vi "FH5dataout.vi"() -> ()   [LabVIEW 2020]
uses:
  Velocimetro.ctl
  ContaGiro.ctl
panel:
  out "RPM x Speed":sgl[][](graph)
  out "Numeric 2":sgl format="%_4f"
  out "Numeric":sgl format="%_3g"
  out "Velocidade Km/h":T1 scale=0.0..300.0
  out "RPM":T2 scale=0.0..8.0
  in  "Stop Button":bool
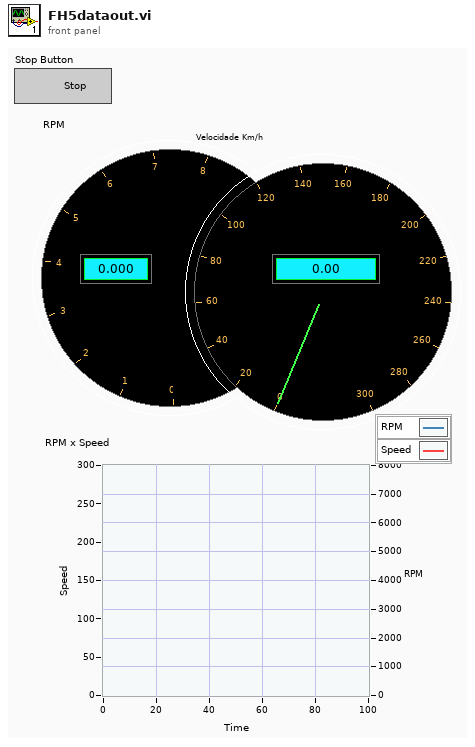
[diagram p1: front panel]
types:
  T1 = typedef "Velocimetro.ctl" = dbl
  T2 = typedef "ContaGiro.ctl" = dbl
  T3 = cluster{"IsRaceOn":i32, "TimestampMS":u32, "EngineMaxRpm":sgl, "EngineIdleRpm":sgl, "CurrentEngineRpm":sgl, "AccelerationX":sgl, "AccelerationY":sgl, "AccelerationZ":sgl, "VelocityX":sgl, "VelocityY":sgl, "VelocityZ":sgl, "AngularVelocityX":sgl, "AngularVelocityY":sgl, "AngularVelocityZ":sgl, "Yaw":sgl, "Pitch":sgl, "Roll":sgl, "NormalizedSuspensionTravelFrontLeft":sgl, "NormalizedSuspensionTravelFrontRight":sgl, "NormalizedSuspensionTravelRearLeft":sgl, "NormalizedSuspensionTravelRearRight":sgl, "TireSlipRatioFrontLeft":sgl, "TireSlipRatioFrontRight":sgl, "TireSlipRatioRearLeft":sgl, "TireSlipRatioRearRight":sgl, "WheelRotationSpeedFrontLeft":sgl, "WheelRotationSpeedFrontRight":sgl, "WheelRotationSpeedRearLeft":sgl, "WheelRotationSpeedRearRight":sgl, "WheelOnRumbleStripFrontLeft":i32, "WheelOnRumbleStripFrontRight":i32, "WheelOnRumbleStripRearLeft":i32, "WheelOnRumbleStripRearRight":i32, "WheelInPuddleDepthFrontLeft":sgl, "WheelInPuddleDepthFrontRight":sgl, "WheelInPuddleDepthRearLeft":sgl, "WheelInPuddleDepthRearRight":sgl, "SurfaceRumbleFrontLeft":sgl, "SurfaceRumbleFrontRight":sgl, "SurfaceRumbleRearLeft":sgl, "SurfaceRumbleRearRight":sgl, "TireSlipAngleFrontLeft":sgl, "TireSlipAngleFrontRight":sgl, "TireSlipAngleRearLeft":sgl, "TireSlipAngleRearRight":sgl, "TireCombinedSlipFrontLeft":sgl, "TireCombinedSlipFrontRight":sgl, "TireCombinedSlipRearLeft":sgl, "TireCombinedSlipRearRight":sgl, "SuspensionTravelMetersFrontLeft":sgl, "SuspensionTravelMetersFrontRight":sgl, "SuspensionTravelMetersRearLeft":sgl, "SuspensionTravelMetersRearRight":sgl, "CarOrdinal":i32, "CarClass":i32, "CarPerformanceIndex":i32, "DrivetrainType":i32, "NumCylinders":i32, "HorizonPlaceholderUKNDATA":u32, "HorizonPlaceholderUKNDATA1":u32, "HorizonPlaceholderUKNDATA2":u32, "PositionX":sgl, "PositionY":sgl, "PositionZ":sgl, "Speed":sgl, "Power":sgl, "Torque":sgl, "TireTempFrontLeft":sgl, "TireTempFrontRight":sgl, "TireTempRearLeft":sgl, "TireTempRearRight":sgl, "Boost":sgl, "Fuel":sgl, "DistanceTraveled":sgl, "BestLap":sgl, "LastLap":sgl, "CurrentLap":sgl, "CurrentRaceTime":sgl, "LapNumber":u16, "RacePosition":u8, "Accel":u8, "Brake":u8, "Clutch":u8, "HandBrake":u8, "Gear":u8, "Steer":i8, "NormalizedDrivingLine":i8, "NormalizedAIBrakeDifference":i8, "UNKNOWNDATA4":u8}
  T4 = enum16{"big-endian, network order", "native, host order", "little-endian"}
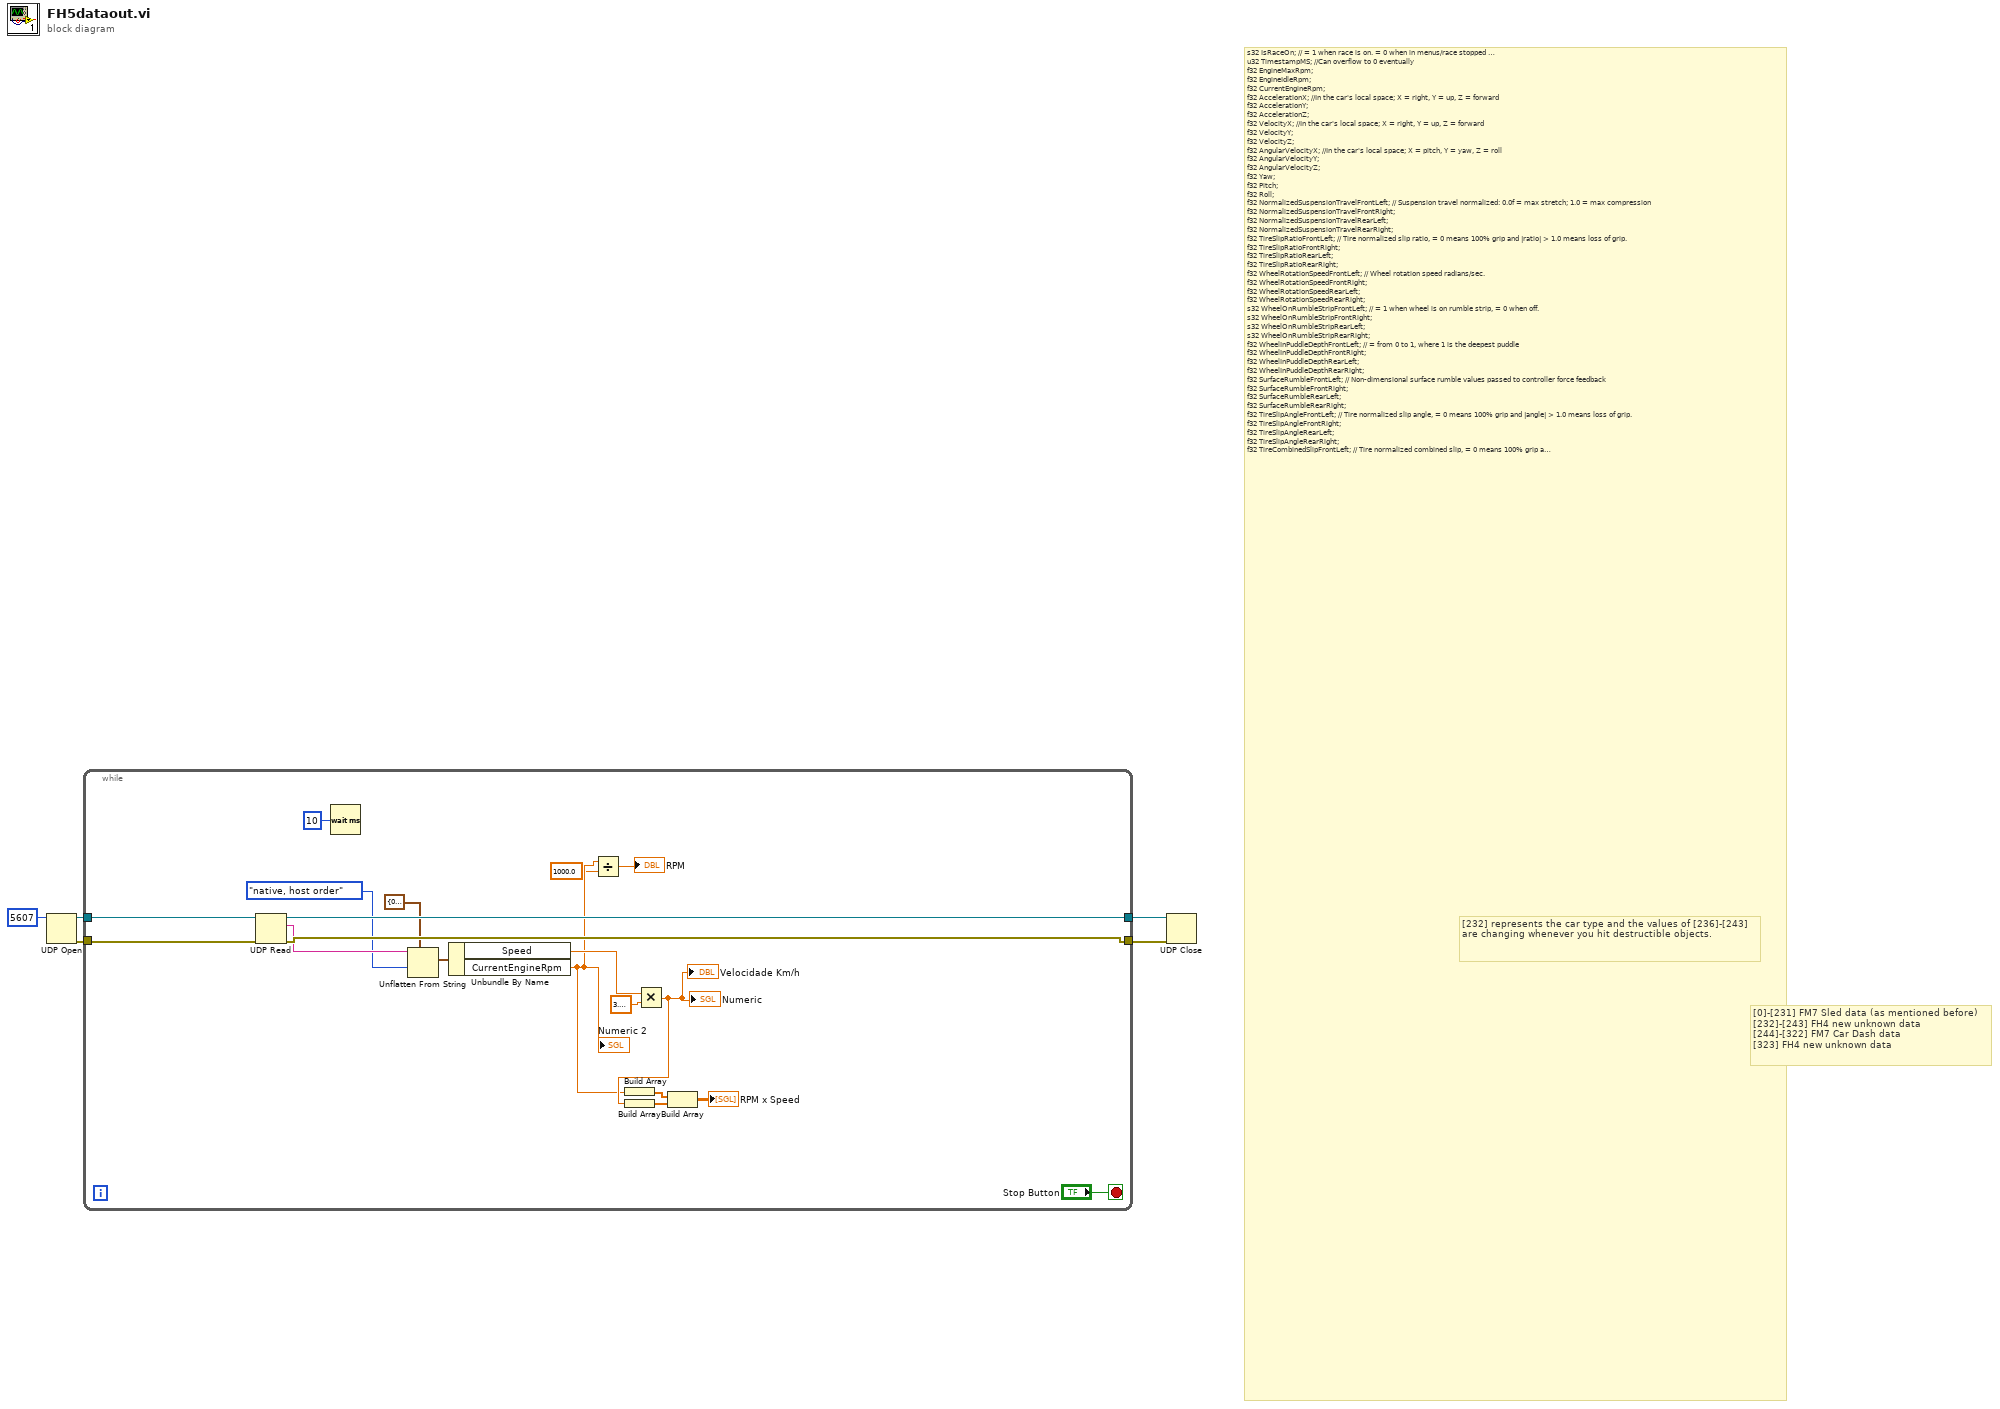
[diagram p0: block diagram]
diagram:
  # "[0]-[231] FM7 Sled data (as mentioned before)\n[232]-[243] FH4 new unknown data\n[244]-[322] FM7 Car Dash data\n[323] FH4 new unknown data"
  # "s32 IsRaceOn; // = 1 when race is on. = 0 when in menus/race stopped …\nu32 TimestampMS; //Can overflow to 0 eventually\nf32 EngineMaxRpm;\nf32 EngineIdleRpm;\nf32 CurrentEngineRpm;\nf32 AccelerationX; //In the car's local space; X = right, Y = up, Z = forward\nf32 AccelerationY;\nf32 AccelerationZ;\nf32 VelocityX; //In the car's local space; X = right, Y = up, Z = forward\nf32 VelocityY;\nf32 VelocityZ;\nf32 AngularVelocityX; //In the car's local space; X = pitch, Y = yaw, Z = roll\nf32 AngularVelocityY;\nf32 AngularVelocityZ;\nf32 Yaw;\nf32 Pitch;\nf32 Roll;\nf32 NormalizedSuspensionTravelFrontLeft; // Suspension travel normalized: 0.0f = max stretch; 1.0 = max compression\nf32 NormalizedSuspensionTravelFrontRight;\nf32 NormalizedSuspensionTravelRearLeft;\nf32 NormalizedSuspensionTravelRearRight;\nf32 TireSlipRatioFrontLeft; // Tire normalized slip ratio, = 0 means 100% grip and |ratio| > 1.0 means loss of grip.\nf32 TireSlipRatioFrontRight;\nf32 TireSlipRatioRearLeft;\nf32 TireSlipRatioRearRight;\nf32 WheelRotationSpeedFrontLeft; // Wheel rotation speed radians/sec.\nf32 WheelRotationSpeedFrontRight;\nf32 WheelRotationSpeedRearLeft;\nf32 WheelRotationSpeedRearRight;\ns32 WheelOnRumbleStripFrontLeft; // = 1 when wheel is on rumble strip, = 0 when off.\ns32 WheelOnRumbleStripFrontRight;\ns32 WheelOnRumbleStripRearLeft;\ns32 WheelOnRumbleStripRearRight;\nf32 WheelInPuddleDepthFrontLeft; // = from 0 to 1, where 1 is the deepest puddle\nf32 WheelInPuddleDepthFrontRight;\nf32 WheelInPuddleDepthRearLeft;\nf32 WheelInPuddleDepthRearRight;\nf32 SurfaceRumbleFrontLeft; // Non-dimensional surface rumble values passed to controller force feedback\nf32 SurfaceRumbleFrontRight;\nf32 SurfaceRumbleRearLeft;\nf32 SurfaceRumbleRearRight;\nf32 TireSlipAngleFrontLeft; // Tire normalized slip angle, = 0 means 100% grip and |angle| > 1.0 means loss of grip.\nf32 TireSlipAngleFrontRight;\nf32 TireSlipAngleRearLeft;\nf32 TireSlipAngleRearRight;\nf32 TireCombinedSlipFrontLeft; // Tire normalized combined slip, = 0 means 100% grip and |slip| > 1.0 means loss of grip.\nf32 TireCombinedSlipFrontRight;\nf32 TireCombinedSlipRearLeft;\nf32 TireCombinedSlipRearRight;\nf32 SuspensionTravelMetersFrontLeft; // Actual suspension travel in meters\nf32 SuspensionTravelMetersFrontRight;\nf32 SuspensionTravelMetersRearLeft;\nf32 SuspensionTravelMetersRearRight;\ns32 CarOrdinal; //Unique ID of the car make/model\ns32 CarClass; //Between 0 (D -- worst cars) and 7 (X class -- best cars) inclusive\ns32 CarPerformanceIndex; //Between 100 (slowest car) and 999 (fastest car) inclusive\ns32 DrivetrainType; //Corresponds to EDrivetrainType; 0 = FWD, 1 = RWD, 2 = AWD\ns32 NumCylinders; //Number of cylinders in the engine\nhzn HorizonPlaceholder; // unknown FH4 values\nf32 PositionX;\nf32 PositionY;\nf32 PositionZ;\nf32 Speed; // meters per second\nf32 Power; // watts\nf32 Torque; // newton meter\nf32 TireTempFrontLeft;\nf32 TireTempFrontRight;\nf32 TireTempRearLeft;\nf32 TireTempRearRight;\nf32 Boost;\nf32 Fuel;\nf32 DistanceTraveled;\nf32 BestLap;\nf32 LastLap;\nf32 CurrentLap;\nf32 CurrentRaceTime;\nu16 LapNumber;\nu8 RacePosition;\nu8 Accel;\nu8 Brake;\nu8 Clutch;\nu8 HandBrake;\nu8 Gear;\ns8 Steer;\ns8 NormalizedDrivingLine;\ns8 NormalizedAIBrakeDifference;"
  # "[232] represents the car type and the values of [236]-[243] \nare changing whenever you hit destructible objects."
  n1 = UDP Open(11:u16 5607 ("port")) -> (port=w5:refnum<k16>, 0:w4:errorcluster)  [unwired: 4 in, 1 out]
  n2 = while {
    tunnel: w5 -> [w24]
    tunnel: [w22] -> w3
    tunnel: w4 -> [w23]
    tunnel: [w21] -> w2
    stop <- "Stop Button" stop-if-true
    n3 = UDP Read(connection ID=w24, 8:w23) -> (data out=w19:string, error out=w21:errorcluster, 3:w22:refnum<k16>)  [unwired: 2 in, 2 out]
    n4 = Wait (ms)(milliseconds to wait=u32 10) -> ()  [unwired: 1 out]
    n5 = Unflatten From String(type=T3 {"IsRaceOn"=0, "TimestampMS"=0, "EngineMaxRpm"=0.0, "EngineIdleRpm"=0.0, "CurrentEngineRpm"=0.0, "AccelerationX"=0.0, "AccelerationY"=0.0, "AccelerationZ"=0.0, "VelocityX"=0.0, "VelocityY"=0.0, "VelocityZ"=0.0, "AngularVelocityX"=0.0, "AngularVelocityY"=0.0, "AngularVelocityZ"=0.0, "Yaw"=0.0, "Pitch"=0.0, "Roll"=0.0, "NormalizedSuspensionTravelFrontLeft"=0.0, "NormalizedSuspensionTravelFrontRight"=0.0, "NormalizedSuspensionTravelRearLeft"=0.0, "NormalizedSuspensionTravelRearRight"=0.0, "TireSlipRatioFrontLeft"=0.0, "TireSlipRatioFrontRight"=0.0, "TireSlipRatioRearLeft"=0.0, "TireSlipRatioRearRight"=0.0, "WheelRotationSpeedFrontLeft"=0.0, "WheelRotationSpeedFrontRight"=0.0, "WheelRotationSpeedRearLeft"=0.0, "WheelRotationSpeedRearRight"=0.0, "WheelOnRumbleStripFrontLeft"=0, "WheelOnRumbleStripFrontRight"=0, "WheelOnRumbleStripRearLeft"=0, "WheelOnRumbleStripRearRight"=0, "WheelInPuddleDepthFrontLeft"=0.0, "WheelInPuddleDepthFrontRight"=0.0, "WheelInPuddleDepthRearLeft"=0.0, "WheelInPuddleDepthRearRight"=0.0, "SurfaceRumbleFrontLeft"=0.0, "SurfaceRumbleFrontRight"=0.0, "SurfaceRumbleRearLeft"=0.0, "SurfaceRumbleRearRight"=0.0, "TireSlipAngleFrontLeft"=0.0, "TireSlipAngleFrontRight"=0.0, "TireSlipAngleRearLeft"=0.0, "TireSlipAngleRearRight"=0.0, "TireCombinedSlipFrontLeft"=0.0, "TireCombinedSlipFrontRight"=0.0, "TireCombinedSlipRearLeft"=0.0, "TireCombinedSlipRearRight"=0.0, "SuspensionTravelMetersFrontLeft"=0.0, "SuspensionTravelMetersFrontRight"=0.0, "SuspensionTravelMetersRearLeft"=0.0, "SuspensionTravelMetersRearRight"=0.0, "CarOrdinal"=0, "CarClass"=0, "CarPerformanceIndex"=0, "DrivetrainType"=0, "NumCylinders"=0, "HorizonPlaceholderUKNDATA"=0, "HorizonPlaceholderUKNDATA1"=0, "HorizonPlaceholderUKNDATA2"=0, "PositionX"=0.0, "PositionY"=0.0, "PositionZ"=0.0, "Speed"=0.0, "Power"=0.0, "Torque"=0.0, "TireTempFrontLeft"=0.0, "TireTempFrontRight"=0.0, "TireTempRearLeft"=0.0, "TireTempRearRight"=0.0, "Boost"=0.0, "Fuel"=0.0, "DistanceTraveled"=0.0, "BestLap"=0.0, "LastLap"=0.0, "CurrentLap"=0.0, "CurrentRaceTime"=0.0, "LapNumber"=0, "RacePosition"=0, "Accel"=0, "Brake"=0, "Clutch"=0, "HandBrake"=0, "Gear"=0, "Steer"=0, "NormalizedDrivingLine"=0, "NormalizedAIBrakeDifference"=0, "UNKNOWNDATA4"=0}, binary string=w19, byte order (0:big-endian, network order)=T4."native, host order") -> (value=w15:T3)  [unwired: 2 in, 2 out]
    n6 = Unbundle By Name(w15) -> ("Speed"=w14:sgl, "CurrentEngineRpm"=w7:sgl)
    "Numeric 2" <- w7
    n7 = Divide(x=w7, y=sgl 1000.0) -> (x/y=→"RPM":sgl)
    n8 = Build Array(w7) -> (w12:sgl[])
    n9 = Multiply(x=w14, y=sgl 3.6) -> (x*y=w13:sgl)
    "Velocidade Km/h" <- w13
    "Numeric" <- w13
    n10 = Build Array(w13) -> (w11:sgl[])
    n11 = Build Array(w12, w11) -> (→"RPM x Speed":sgl[][])
  }
  n12 = UDP Close(connection ID=w3, 8:w2) -> ()  [unwired: 2 out]
